vi "TDC_freezeBuffers.vi"(8 "Error In":errorcluster, 11 "Freeze":bool) -> (0 "Error Out":errorcluster)   [LabVIEW 2011]
uses:
  dist/userlib/lib/tdcbase.dll
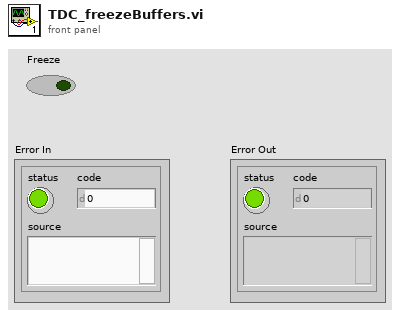
[diagram p1: front panel]
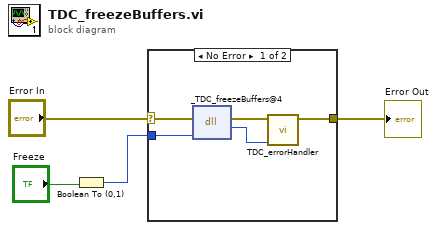
[diagram p0: block diagram]
diagram:
  n1 = Boolean To (0,1)(Boolean="Freeze") -> (0, 1=w1:i16)
  n2 = case shown="No Error" "Error In" {
    selector: "Error In" -> [w9 w10]
    tunnel: [w6 w10] -> w3
    tunnel: w1 -> [w5 _]
    frame No Error {
      n3 = dll-call lib="C:/nh/projekt/spmctrl/dist/userlib/lib/tdcbase.dll" fn="_TDC_freezeBuffers@4"(error in=w9, "freeze"=w5) -> (error out=w8:errorcluster, "return type"=w7:i32)  [unwired: 3 in, 1 out]
      n4 = call "TDC_errorHandler.vi"("quTAU Return Code"=w7, "Error In"=w8) -> ("Error Out"=w6:errorcluster)  [unwired: 9 in]
    }
    frame Error {
    }
  }
  "Error Out" <- w3
